vi "Hub Write.vi"(8 "error in (no error)":errorcluster, 9 "hub port":u64=2, 10 "data in":string, 11 "RP Communicator in":refnum<class "RP Communicator.lvclass">) -> (0 "error out":errorcluster, 3 "RP Communicator out":refnum<class "RP Communicator.lvclass">)   [LabVIEW 2024, in "RP Communicator.lvclass"]
uses:
  RP Communicator.lvclass
  RP Communicator.lvclass/RP Communicator.ctl
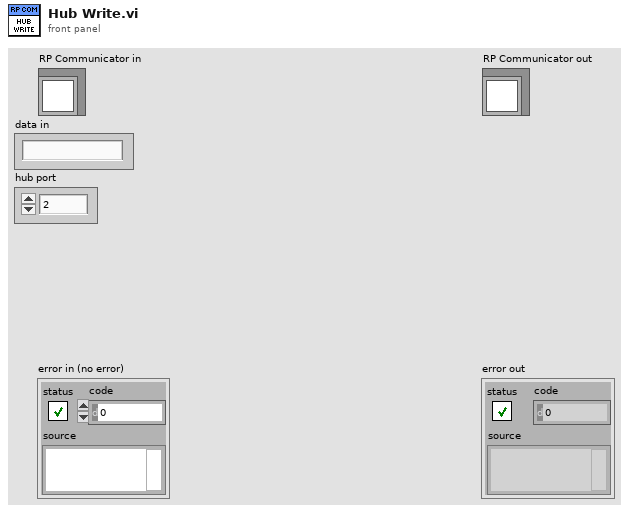
[diagram p1: front panel]
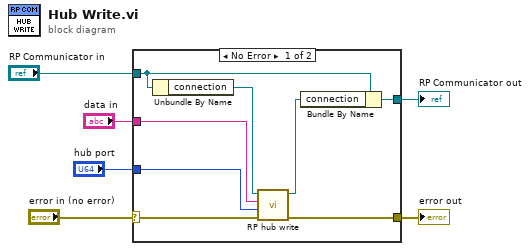
[diagram p0: block diagram]
diagram:
  n1 = case shown="No Error" "error in (no error)" {
    selector: "error in (no error)" -> [w9 w16]
    tunnel: [w10 w16] -> w5
    tunnel: [w12 w15] -> w3
    tunnel: "RP Communicator in" -> [w14 w15]
    tunnel: "data in" -> [w8 _]
    tunnel: "hub port" -> [w7 _]
    frame No Error {
      n2 = Unbundle By Name(w14) -> ("connection"=w13:refnum<k5>)
      n3 = call "RP hub write.vi"("Error In"=w9, "hub port"=w7, "data in"=w8, "connection ID"=w13) -> ("Error Out"=w10:errorcluster, "connection ID out"=w11:refnum<k5>)  [unwired: 6 in]
      n4 = Bundle By Name(cluster=w14, "connection"=w11) -> (w12:refnum<class "RP Communicator.lvclass">)
    }
    frame Error {
    }
  }
  "error out" <- w5
  "RP Communicator out" <- w3
